vi "Analog Voltage DAQ Setup.vi"(0 "task in":refnum<k21>, 5 "physical channels":tag, 11 "error in":errorcluster, 12 "Sample Rate":dbl=1000.0 format="%0.2f", 13 "samples per channel":i32=1) -> (4 "task out":refnum<k21>, 15 "error out":errorcluster)   [LabVIEW 2016]
uses:
  <vilib>/DAQmx/create/channels.llb/DAQmx Create Channel (AI-Voltage-Basic).vi
  <vilib>/DAQmx/configure/timing.llb/DAQmx Timing (Sample Clock).vi
panel:
  in  "minimum value":dbl format="%0.2f"
  in  "input terminal configuration":i32(ring)=10083 items=["Default"=-1, "RSE"=10083, "NRSE"=10078, "Differential"=10106, "Pseudodifferential"=12529]
  in  "maximum value":dbl=1.0 format="%0.2f"
  in  "sample mode":i32(ring)=10123 items=["Finite Samples"=10178, "Continuous Samples"=10123, "Hardware Timed Single Point"=12522]
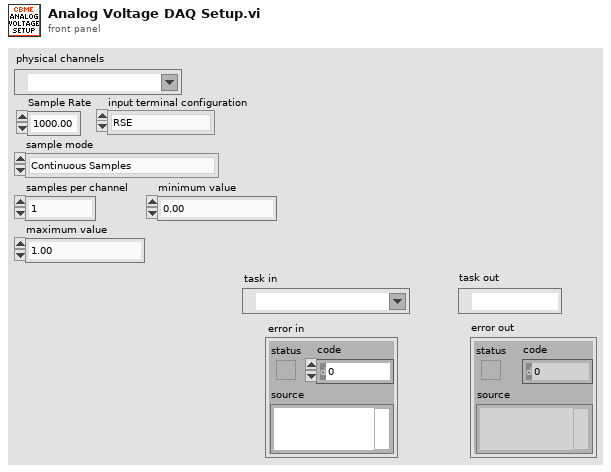
[diagram p1: front panel]
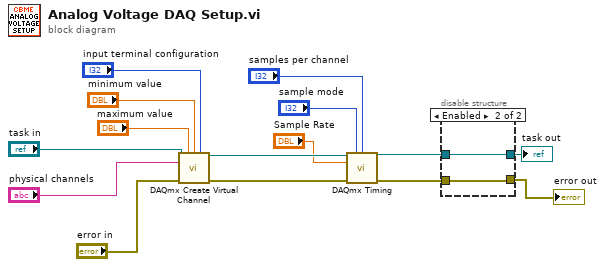
[diagram p0: block diagram]
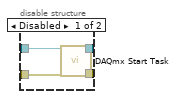
[diagram p2: hidden frame]
diagram:
  n1 = call-poly <vilib>:"DAQmx Create Virtual Channel.vi"("task in"="task in", "maximum value"="maximum value", "minimum value"="minimum value", "input terminal configuration"="input terminal configuration", "physical channels"="physical channels", "error in"="error in") -> ("task out"=w14:refnum<k21>, "error out"=w10:errorcluster)  [unwired: 8 in]
  n2 = call-poly <vilib>:"DAQmx Timing.vi"("task/channels in"=w14, "sample mode"="sample mode", "samples per channel"="samples per channel", "rate"="Sample Rate", "error in"=w10) -> ("task out"=w9:refnum<k21>, "error out"=w8:errorcluster)  [unwired: 9 in]
  n3 = disable-structure shown="Enabled" {
    disable-tunnel: w9 -> [w19 w21]
    disable-tunnel: w8 -> [w18 w20]
    disable-tunnel: [w17 w21] -> w7
    disable-tunnel: [w16 w20] -> w6
    frame Disabled {
      n4 = call <vilib>:"DAQmx Start Task.vi"("task/channels in"=w19, "error in"=w18) -> ("task out"=w17:refnum<k21>, "error out"=w16:errorcluster)  [unwired: 12 in]
    }
    frame Enabled {
    }
  }
  "task out" <- w7
  "error out" <- w6
